vi "Set Injection.vi"(8 "error in (no error)":errorcluster, 9 "Enable":bool, 10 "Value":T1, 11 "Fault-Injection_Boolean in":refnum<class "Fault-Injection_Boolean.lvclass">) -> (0 "error out":errorcluster, 3 "Fault-Injection_Boolean out":refnum<class "Fault-Injection_Boolean.lvclass">)   [LabVIEW 2021, in "Fault-Injection_Boolean.lvclass"]
uses:
  Fault-Injection_Boolean.lvclass
  Fault-Injection_Boolean.lvclass/Fault-Injection_Boolean.ctl
  Support/Value Type.ctl
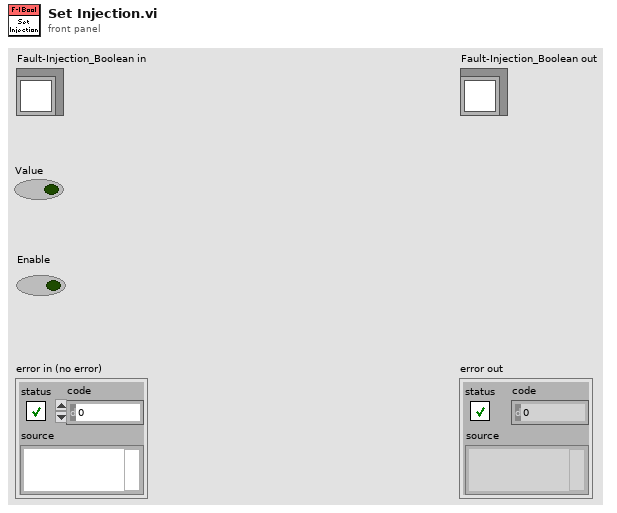
[diagram p1: front panel]
types:
  T1 = typedef "Fault-Injection_Boolean.lvclass/Value Type.ctl" = bool
  T2 = typedef "Fault-Injection_Boolean.lvclass/DVR Type.ctl" = cluster{"Enable":bool, "Injected Value":T1, "Value":refnum<class "Abs_Boolean.lvclass">}
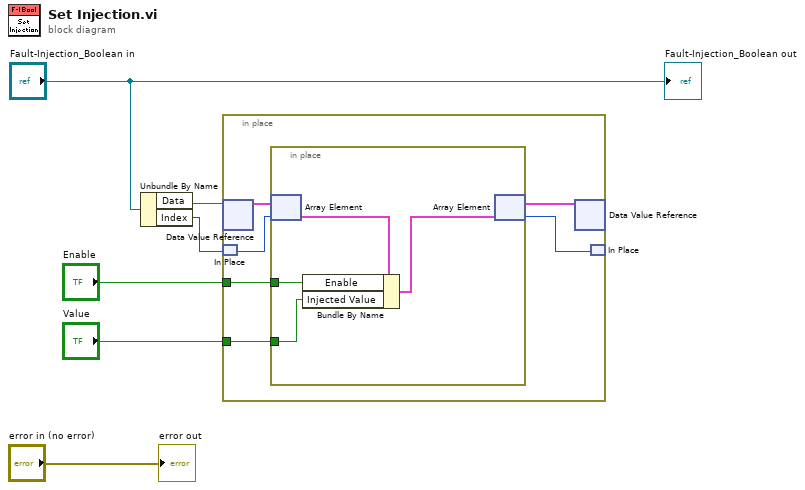
[diagram p0: block diagram]
diagram:
  n1 = Unbundle By Name("Fault-Injection_Boolean in") -> ("Data"=w5:refnum<data-value>, "Index"=w4:i32)
  n2 = in-place {
    in-place-border: "Enable" -> [w8]
    in-place-border: "Value" -> [w7]
    n3 = in-place-dvr #1(w5) -> (w12:T2[])  [unwired: 1 out]
    n4 = in-place-match #2(w4) -> (w10:i32)
    n5 = in-place {
      in-place-border: w8 -> [w14]
      in-place-border: w7 -> [w13]
      n6 = in-place-array #3(w12, w10) -> (w16:T2)
      n7 = Bundle By Name(cluster=w16, "Enable"=w14, "Injected Value"=w13) -> (w15:T2)
      n8 = in-place-array #3(w15) -> (w11:T2[], w9:i32)
    }
    n9 = in-place-dvr #1(w11) -> ()  [unwired: 2 out]
    n10 = in-place-match #2(w9) -> ()  [unwired: 1 out]
  }
  "error out" <- "error in (no error)"
  "Fault-Injection_Boolean out" <- "Fault-Injection_Boolean in"
